vi "Serialize.vi"(8 "error in (no error)":errorcluster, 10 "Item Info":refnum<class "XML Node.lvclass">, 11 "Build Package Item in":refnum<class "Build Package Item.lvclass">) -> (0 "error out":errorcluster, 2 "Serialization Version":string)   [LabVIEW 2019, in "VIPM.lvlib" / "Build Package Item.lvclass"]
uses:
  Build Package Item.lvclass
  libs/Solution.lvlibp/Solution/XML Reader/XML Node.lvclass
  Build Package Item.lvclass/Build Package Item.ctl
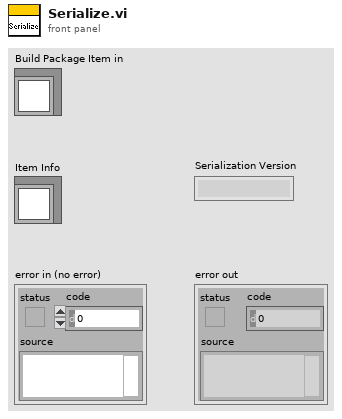
[diagram p1: front panel]
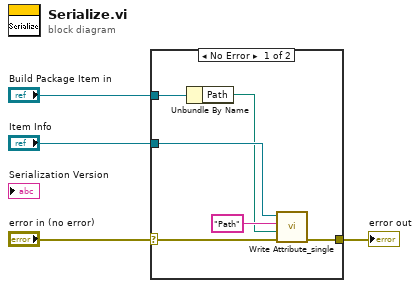
[diagram p0: block diagram]
diagram:
  n1 = case shown="No Error" "error in (no error)" {
    selector: "error in (no error)" -> [w9 w11]
    tunnel: "Item Info" -> [w10 _]
    tunnel: [w8 w11] -> w2
    tunnel: "Build Package Item in" -> [w6 _]
    frame No Error {
      n2 = Unbundle By Name(w6) -> ("Path"=w5:path)
      n3 = call "Write Attribute_single.vi"("error in (no error)"=w9, "Value"=w5, "Name"="Path", "XML Node in"=w10) -> ("error out"=w8:errorcluster)  [unwired: 7 in]
    }
    frame Error {
    }
  }
  "error out" <- w2
